vi "EncodersGyroToXY-254.vi"(6 "Reset":bool, 9 "Angle (degrees)":dbl, 10 "Right Distance":dbl, 11 "Left Distance":dbl) -> (3 "Location":cluster{"X":dbl, "Y":dbl})   [LabVIEW 2018]
uses:
  <vilib>/Analysis/coordinate.llb/2D Cartesian Coordinate Rotation (Scalar).vi
  <vilib>/Analysis/NI_AALPro.lvlib
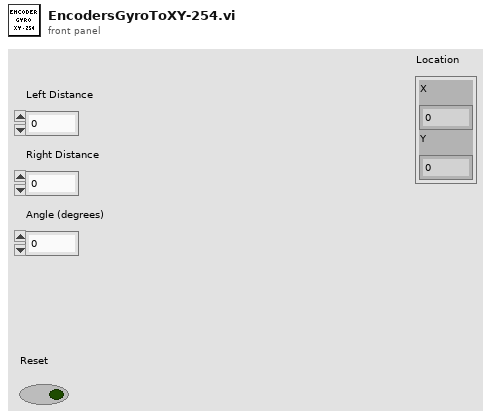
[diagram p1: front panel]
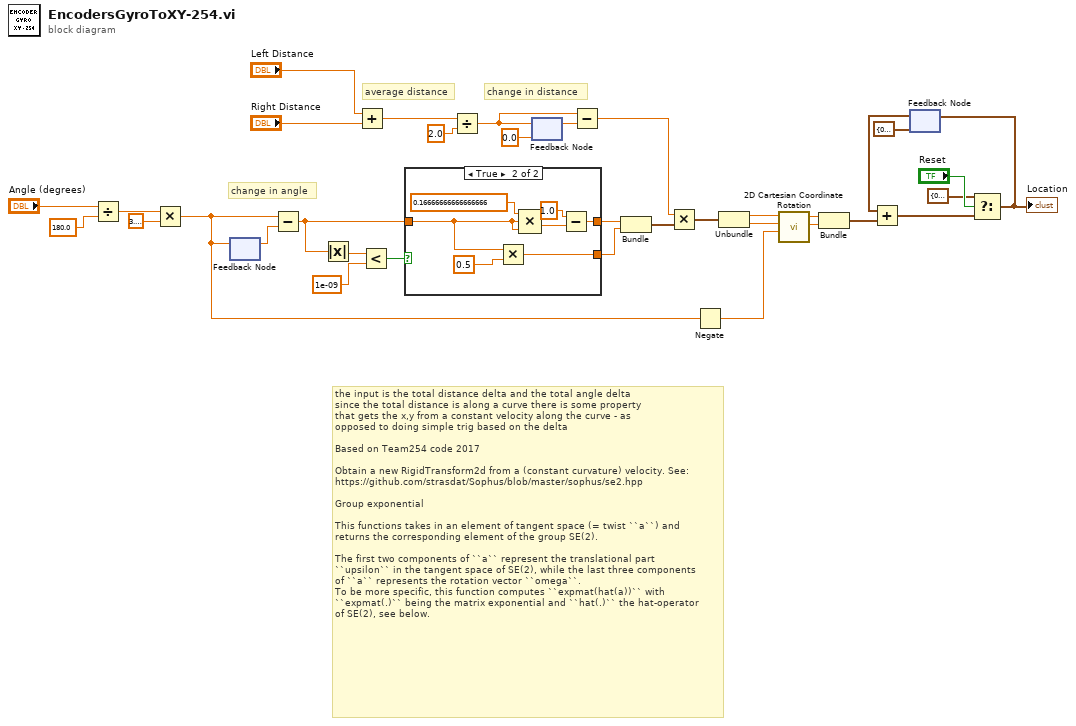
[diagram p0: block diagram]
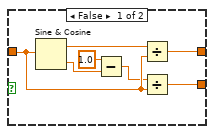
[diagram p2: hidden frame]
diagram:
  # "change in angle"
  # "the input is the total distance delta and the total angle delta\nsince the total distance is along a curve there is some property \nthat gets the x,y from a constant velocity along the curve - as\nopposed to doing simple trig based on the delta\n\nBased on Team254 code 2017\n\nObtain a new RigidTransform2d from a (constant curvature) velocity. See:\nhttps://github.com/strasdat/Sophus/blob/master/sophus/se2.hpp\n\nGroup exponential\n\nThis functions takes in an element of tangent space (= twist ``a``) and\nreturns the corresponding element of the group SE(2).\n\nThe first two components of ``a`` represent the translational part\n``upsilon`` in the tangent space of SE(2), while the last three components\nof ``a`` represents the rotation vector ``omega``.\nTo be more specific, this function computes ``expmat(hat(a))`` with\n``expmat(.)`` being the matrix exponential and ``hat(.)`` the hat-operator\nof SE(2), see below."
  # "change in distance"
  # "average distance"
  n1 = Divide(x="Angle (degrees)", y=180.0) -> (x/y=w3:dbl)
  n2 = Multiply(x=w3, y=3.141592653589793) -> (x*y=w1:dbl)
  n3 = feedback-in #1(w1) -> ()
  n4 = feedback #1() -> (w21:dbl)  [unwired: 1 in]
  n5 = Subtract(x=w1, y=w21) -> (x-y=w17:dbl)
  n6 = Absolute Value(x=w17) -> (abs(x)=w20:dbl)
  n7 = Add(x="Left Distance", y="Right Distance") -> (x+y=w28:dbl)
  n8 = Less?(x=w20, y=1e-09) -> (x < y?=w18:bool)
  n9 = case shown="True" w18 {
    tunnel: w17 -> [w40 w42]
    tunnel: [w36 w43] -> w16
    tunnel: [w35 w47] -> w15
    frame False {
      n10 = Sine & Cosine(0:w40) -> (1:w41:dbl, 2:w38:dbl)
      n11 = Subtract(x=1.0, y=w38) -> (x-y=w37:dbl)
      n12 = Divide(x=w41, y=w40) -> (x/y=w36:dbl)
      n13 = Divide(x=w37, y=w40) -> (x/y=w35:dbl)
    }
    frame True {
      n14 = Multiply(x=w42, y=0.5) -> (x*y=w47:dbl)
      n15 = Compound Arithmetic op=MULTIPLY(0.16666666666666666 ("y"), w42, w42) -> (w46:dbl)
      n16 = Subtract(x=1.0, y=w46) -> (x-y=w43:dbl)
    }
  }
  n17 = Divide(x=w28, y=2.0) -> (x/y=w27:dbl)
  n18 = feedback #2(0.0) -> (w34:dbl)
  n19 = feedback-in #2(w27) -> ()
  n20 = Subtract(x=w27, y=w34) -> (x-y=w13:dbl)
  n21 = Bundle(w16, w15) -> (w14:cluster{dbl, dbl})  [unwired: 1 in]
  n22 = Multiply(x=w13, y=w14) -> (x*y=w11:cluster{dbl, dbl})
  n23 = Negate(x=w1) -> (-x=w12:dbl)
  n24 = Unbundle(w11) -> (w10:dbl, w9:dbl)
  n25 = call-poly <vilib>:"2D Cartesian Coordinate Rotation.vi"("theta"=w12, "y"=w9, "x"=w10) -> ("y out"=w7:dbl, "x out"=w8:dbl)  [unwired: 6 in, 1 out]
  n26 = Bundle("x out"=w8, "y out"=w7) -> (w6:cluster{"x out":dbl, "y out":dbl})  [unwired: 1 in]
  n27 = feedback #3(cluster{dbl, dbl} {0.0, 0.0}) -> (w32:cluster{dbl, dbl})
  n28 = Add(x=w32, y=w6) -> (x+y=w23:cluster{dbl, dbl})
  n29 = Select(t=cluster{dbl, dbl} {0.0, 0.0}, s="Reset", f=w23) -> (s? t:f=w24:cluster{dbl, dbl})
  "Location" <- w24
  n30 = feedback-in #3(w24) -> ()
